vi "AlliGator Create Phasor Plot Additional Data String.vi"(6 "Average Plot Data (F)":bool, 7 "Include Header String (F)":bool, 8 "error in (no error)":errorcluster, 9 "Calibrated Phasor Plot":T2, 10 "Raw Phasor Plot":T4={"Phasor Plot Name"="", "Raw Phasor Plot"=[], "Phasor Frequency"=0.0, "[Decay Metadata]"=[], "Raw Phasor Plot SDV"=[], "Phasor SDV Options"={"Compute Estimated SDV"=FALSE, "# Replicas"=100, "Use Estimated Average Phasor"=FALSE}, "[Calibration Phasor]"=[]} {"[Decay Metadata]"."# Folds" min=1; "[Decay Metadata]"."ROI Descriptor"."Contours"."Type" items=["No Selection", "Point", "Line", "Rectangle", "Oval", "Polygon", "Freehand Region", "Annulus", "Unused2", "Unused3", "Broken Line", "Freehand Line", "Rotated Rectangle"]}, 11 "Phasor Plot Exported Data":T1) -> (0 "error out":errorcluster, 3 "Phasor Plot Additional Data String":string)   [LabVIEW 2021, in "AlliGator Phasor Graph.lvlib"]
doc: "Creates a string with all the user-requested phasor plot additional data."
uses:
  AlliGator Phasor Graph.lvlib
  AlliGator Raw Phasor Plot Data v4.ctl
  Phasor/Phasor (g, s).ctl
  AlliGator Decay Metadata v3.ctl
  AlliGator Decay Background Subtraction Info.ctl
  AlliGator Baseline Subtraction Method.ctl
  Graphs/XY Graph/XY Graph Plot Shift Parameters.ctl
  Graphs/XY Graph/XY Graph Plot Shift Method.ctl
  AlliGator Decay Extrapolation Parameters.ctl
  Phasor/Phasor Standard Deviation Options.ctl
  Phasor/Calibration Phasor (m, phi).ctl
  AlliGator Phasor Plot Additional Data List.ctl
  Graphs/XY Graph/XY Plot Data.ctl
  AlliGator Phasor Plot Exported Data Selection.ctl
  d5eb63e0-648c-47d6-be91-64ae69301d4e.vi
  28782bb2-77f9-4fec-b09f-3ba0b8238253.vi
  <userlib>/_OpenG.lib/array/array.llb/Filter 1D Array (DBL)__ogtk.vi
  Strings/Strings.lvlib
  Phasor/Phasor.lvlib
  AlliGator Phasor Ratio.lvlib
  Time/Time.lvlib
  <vilib>/Analysis/NI_AALBase.lvlib
  Utilities/Utilities.lvlib
  <userlib>/_OpenG.lib/array/array.llb/openg_array.lvlib
  AlliGator Decay Preprocessing.lvlib
  Graphs/XY Graph/XY Graph Add-Ons.lvlib
panel:
  out "CPU (s)":dbl
  in  "Phasor Plot Exported Data List":T3
  # "see the AlliGator License on the block diagram (Ctrl+E or Window:Show Block Diagram)"
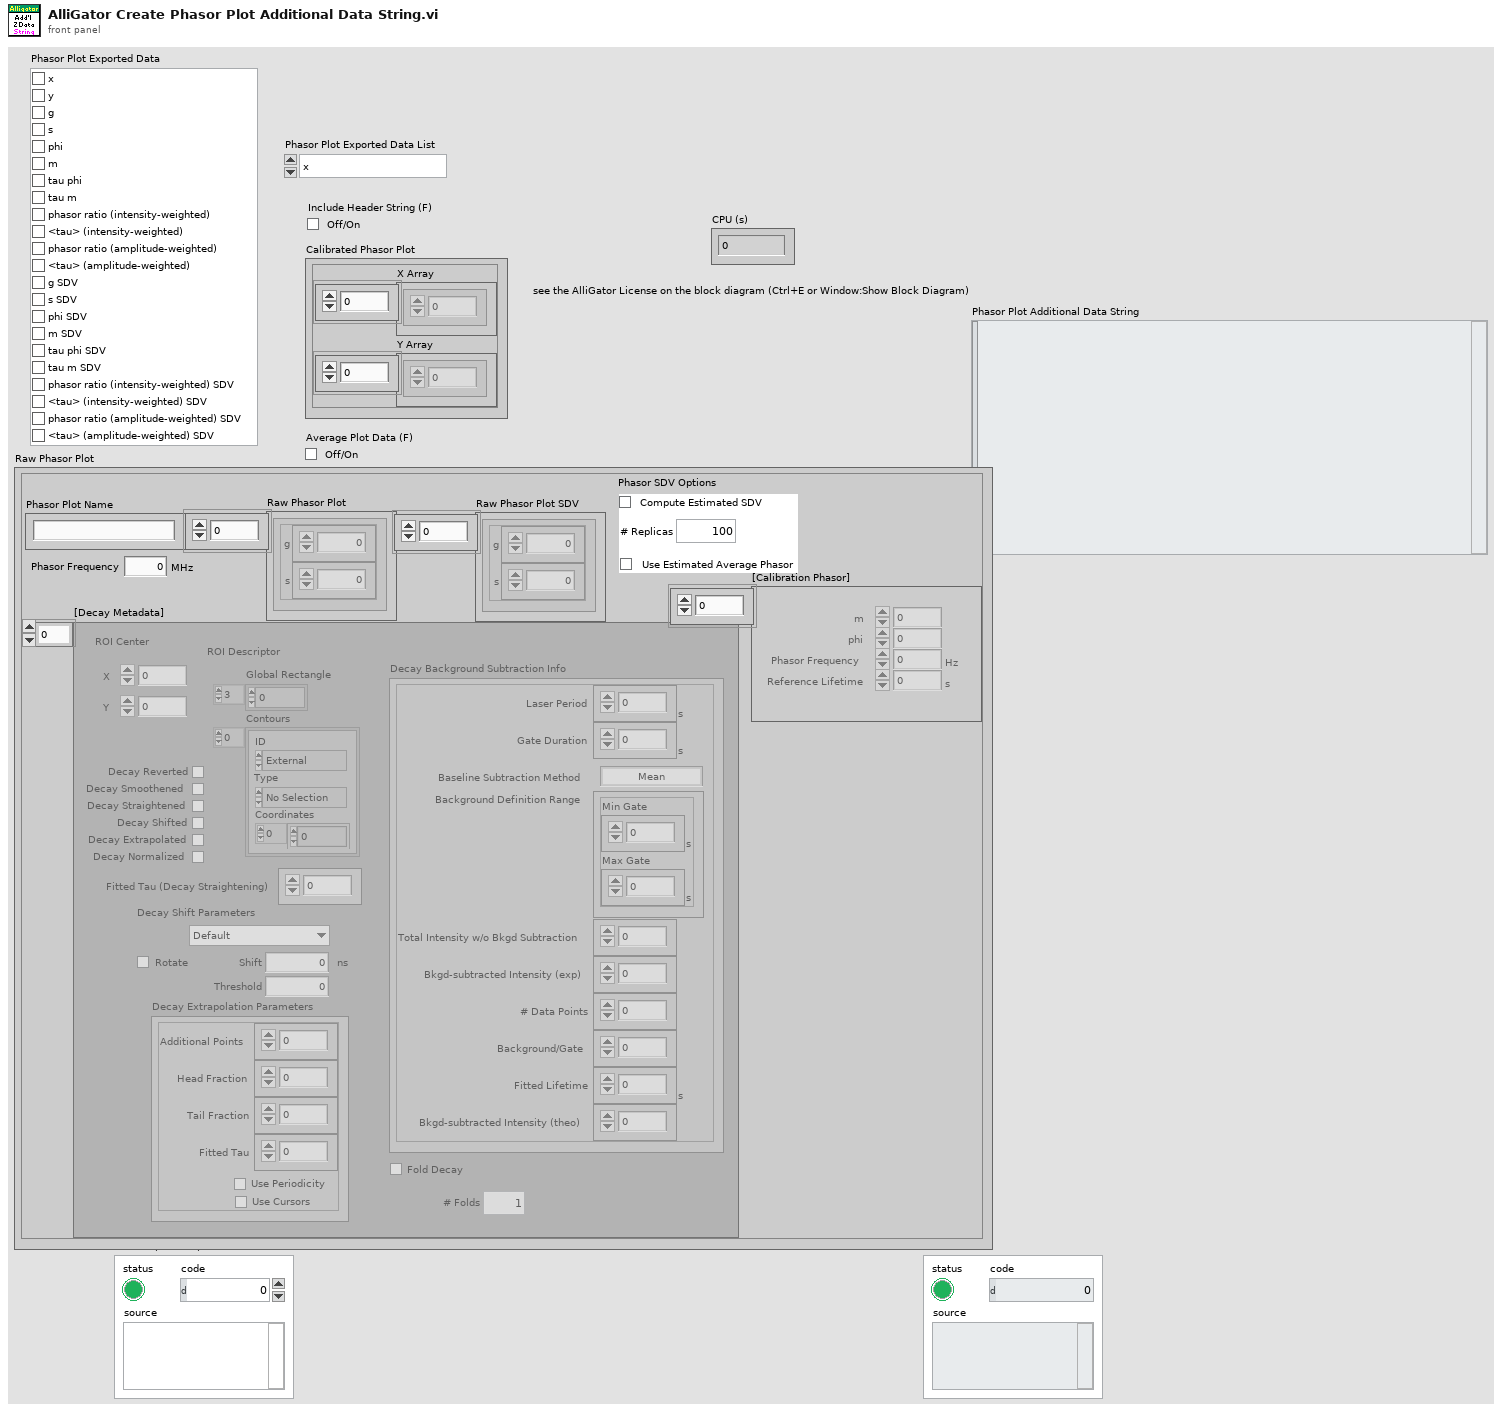
[diagram p1: front panel]
types:
  T1 = typedef "AlliGator Phasor Graph.lvlib/AlliGator Phasor Plot Exported Data Selection.ctl" = cluster{"x":bool, "y":bool, "g":bool, "s":bool, "phi":bool, "m":bool, "tau phi":bool, "tau m":bool, "phasor ratio (intensity-weighted)":bool, "<tau> (intensity-weighted)":bool, "phasor ratio (amplitude-weighted)":bool, "<tau> (amplitude-weighted)":bool, "g SDV":bool, "s SDV":bool, "phi SDV":bool, "m SDV":bool, "tau phi SDV":bool, "tau m SDV":bool, "phasor ratio (intensity-weighted) SDV":bool, "<tau> (intensity-weighted) SDV":bool, "phasor ratio (amplitude-weighted) SDV":bool, "<tau> (amplitude-weighted) SDV":bool}
  T2 = typedef "XY Graph Add-Ons.lvlib/XY Plot Data.ctl" = cluster{"X Array":dbl[], "Y Array":dbl[]}
  T3 = typedef "AlliGator Phasor Graph.lvlib/AlliGator Phasor Plot Additional Data List.ctl" = enum16{"x", "y", "g", "s", "phi", "m", "tau phi", "tau m", "phasor ratio (intensity-weighted)", "<tau> (intensity-weighted)", "phasor ratio (amplitude-weighted)", "<tau> (amplitude-weighted)", "g SDV", "s SDV", "phi SDV", "m SDV", "tau phi SDV", "tau m SDV", "phasor ratio (intensity-weighted) SDV", "<tau> (intensity-weighted) SDV", "phasor ratio (amplitude-weighted) SDV", "<tau> (amplitude-weighted) SDV"}
  T4 = typedef "AlliGator Phasor Graph.lvlib/AlliGator Raw Phasor Plot Data v4.ctl" = cluster{"Phasor Plot Name":string, "Raw Phasor Plot":T5[], "Phasor Frequency":dbl[unit], "[Decay Metadata]":T6[], "Raw Phasor Plot SDV":T5[], "Phasor SDV Options":T13, "[Calibration Phasor]":T14[]}
  T5 = typedef "Phasor.lvlib/Phasor (g, s).ctl" = cluster{"g":dbl, "s":dbl}
  T6 = typedef "AlliGator Phasor Graph.lvlib/AlliGator Decay Metadata v3.ctl" = cluster{"ROI Descriptor":T7, "ROI Center":cluster{"X":i32, "Y":i32}, "Decay Background Subtraction Info":T8, "Decay Reverted":bool, "Decay Smoothened":bool, "Decay Straightened":bool, "Fitted Tau (Decay Straightening)":dbl, "Decay Shift Parameters":T10, "Decay Shifted":bool, "Decay Extrapolated":bool, "Decay Extrapolation Parameters":T12, "Decay Normalized":bool, "Fold Decay":bool, "# Folds":u32}
  T7 = typedef "ROI Descriptor" = cluster{"Global Rectangle":i32[], "Contours":cluster{"ID":enum32{"External", "Internal"}, "Type":u32, "Coordinates":i32[]}[]}
  T8 = typedef "AlliGator Decay Analysis.lvlib/AlliGator Decay Preprocessing.lvlib/AlliGator Decay Background Subtraction Info.ctl" = cluster{"Laser Period":dbl[unit], "Gate Duration":dbl[unit], "Baseline Subtraction Method":T9, "Background Definition Range":cluster{"Min Gate":dbl[unit], "Max Gate":dbl[unit]}, "Total Intensity w/o Bkgd Subtraction":dbl, "Bkgd-subtracted Intensity (exp)":dbl, "# Data Points":i32, "Background/Gate":dbl, "Fitted Lifetime":dbl[unit], "Bkgd-subtracted Intensity (theo)":dbl}
  T9 = typedef "AlliGator Decay Analysis.lvlib/AlliGator Decay Preprocessing.lvlib/AlliGator Baseline Subtraction Method.ctl" = enum16{"Mean", "Min", "Square Gated Single-Exponential", "File", "Constant"}
  T10 = typedef "XY Graph Add-Ons.lvlib/XY Graph Plot Shift Parameters.ctl" = cluster{"Type":T11, "Shift":dbl[unit], "Threshold":dbl, "Rotate":bool}
  T11 = typedef "XY Graph Add-Ons.lvlib/XY Graph Plot Shift Method.ctl" = enum16{"Default", "CFD", "Threshold", "Cross-Correlation"}
  T12 = typedef "AlliGator Decay Analysis.lvlib/AlliGator Decay Preprocessing.lvlib/AlliGator Decay Extrapolation Parameters.ctl" = cluster{"Additional Points":u32, "Head Fraction":dbl, "Fitted Tau":dbl, "Use Periodicity":bool, "Use Cursors":bool, "Tail Fraction":dbl}
  T13 = typedef "Phasor.lvlib/Phasor Standard Deviation Options.ctl" = cluster{"Compute Estimated SDV":bool, "# Replicas":u32, "Use Estimated Average Phasor":bool}
  T14 = typedef "Phasor.lvlib/Calibration Phasor (m, phi).ctl" = cluster{"m":dbl, "phi":dbl, "Phasor Frequency":dbl[unit], "Reference Lifetime":dbl[unit]}
  T15 = cluster{"Numeric Control":dbl, "Numeric Control":dbl}[]
  T16 = typedef "Phasor.lvlib/Phasor (m, phi).ctl" = cluster{"m":dbl, "phi":dbl}
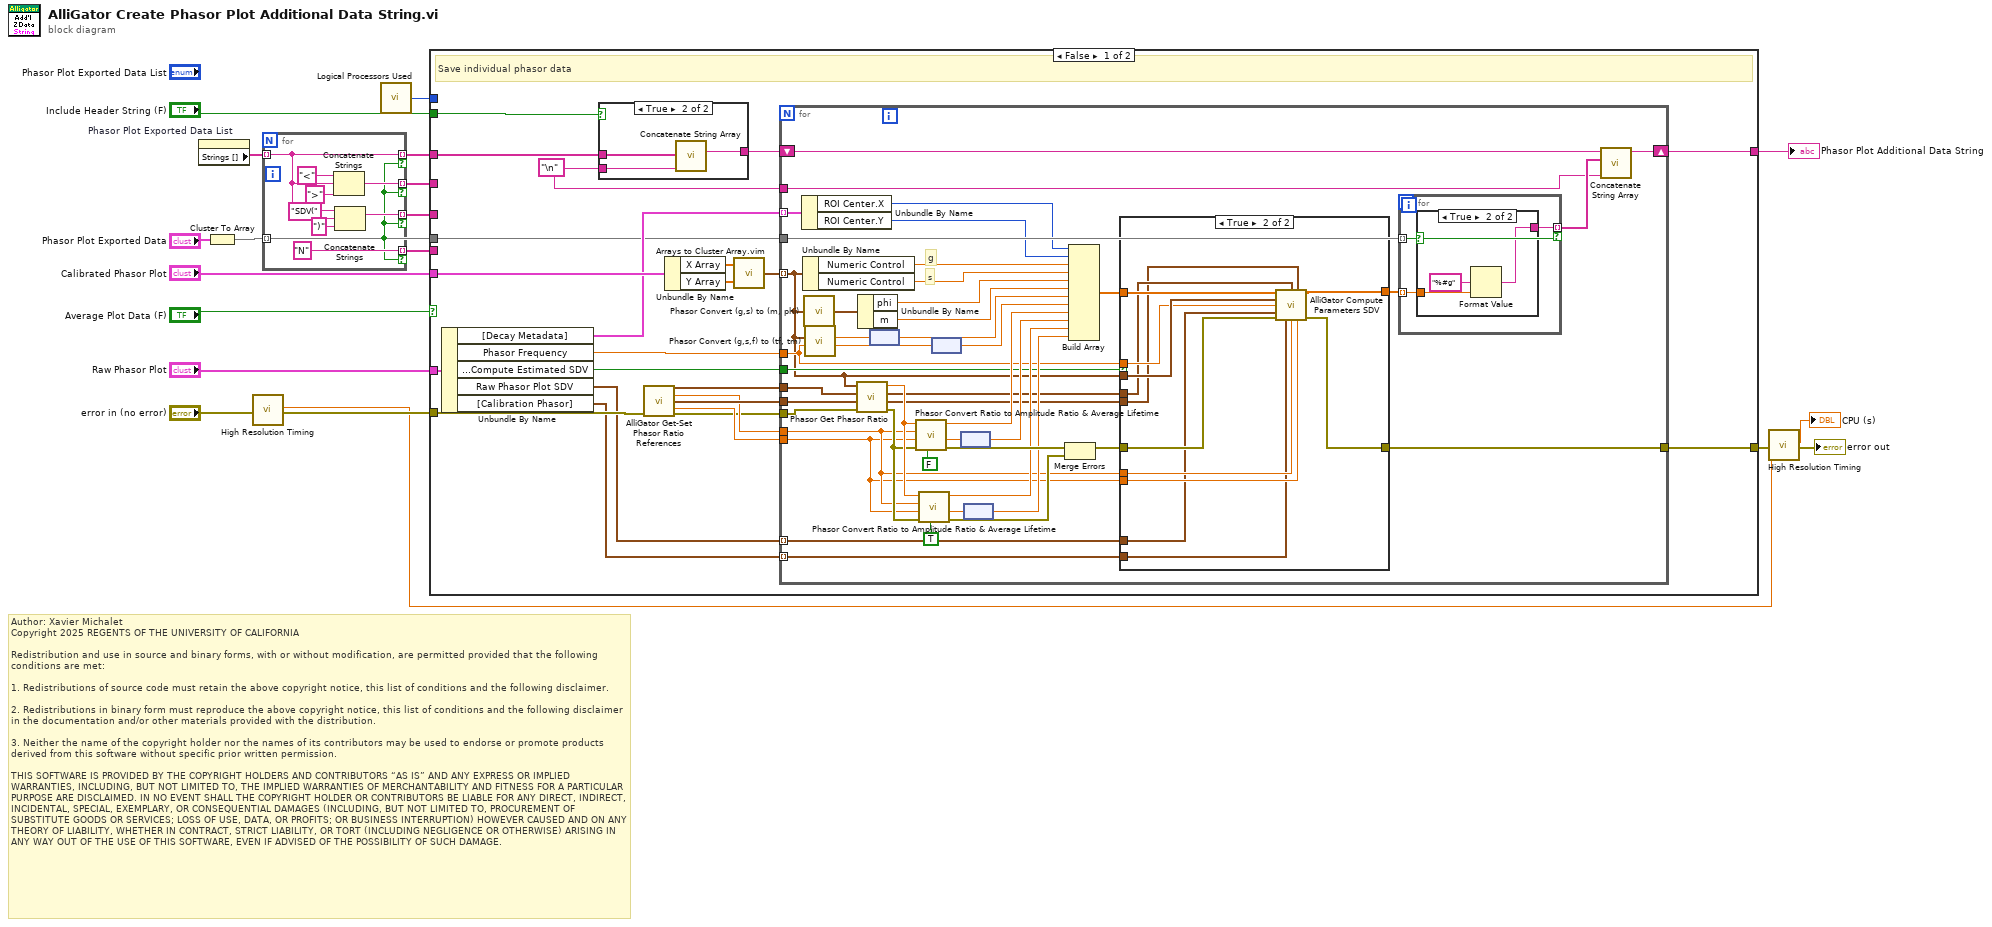
[diagram p0: block diagram]
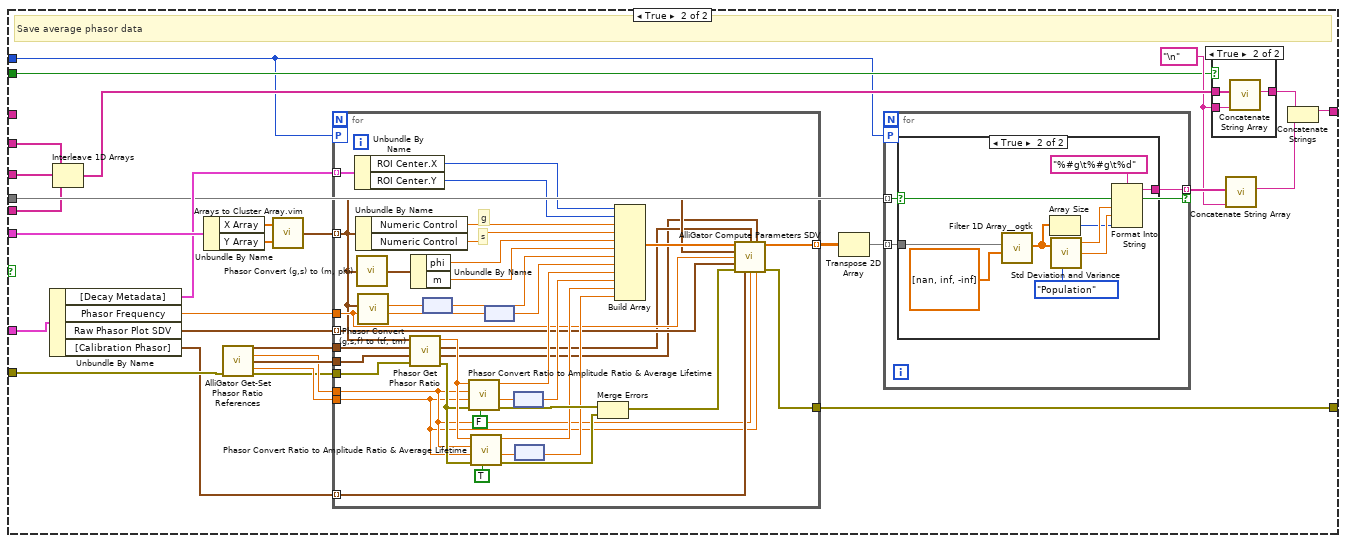
[diagram p5: hidden frame]
diagram:
  # "Author: Xavier Michalet\nCopyright 2025 REGENTS OF THE UNIVERSITY OF CALIFORNIA\n\nRedistribution and use in source and binary forms, with or without modification, are permitted provided that the following conditions are met:\n\n1. Redistributions of source code must retain the above copyright notice, this list of conditions and the following disclaimer.\n\n2. Redistributions in binary form must reproduce the above copyright notice, this list of conditions and the following disclaimer in the documentation and/or other materials provided with the distribution.\n\n3. Neither the name of the copyright holder nor the names of its contributors may be used to endorse or promote products derived from this software without specific prior written permission.\n\nTHIS SOFTWARE IS PROVIDED BY THE COPYRIGHT HOLDERS AND CONTRIBUTORS “AS IS” AND ANY EXPRESS OR IMPLIED WARRANTIES, INCLUDING, BUT NOT LIMITED TO, THE IMPLIED WARRANTIES OF MERCHANTABILITY AND FITNESS FOR A PARTICULAR PURPOSE ARE DISCLAIMED. IN NO EVENT SHALL THE COPYRIGHT HOLDER OR CONTRIBUTORS BE LIABLE FOR ANY DIRECT, INDIRECT, INCIDENTAL, SPECIAL, EXEMPLARY, OR CONSEQUENTIAL DAMAGES (INCLUDING, BUT NOT LIMITED TO, PROCUREMENT OF SUBSTITUTE GOODS OR SERVICES; LOSS OF USE, DATA, OR PROFITS; OR BUSINESS INTERRUPTION) HOWEVER CAUSED AND ON ANY THEORY OF LIABILITY, WHETHER IN CONTRACT, STRICT LIABILITY, OR TORT (INCLUDING NEGLIGENCE OR OTHERWISE) ARISING IN ANY WAY OUT OF THE USE OF THIS SOFTWARE, EVEN IF ADVISED OF THE POSSIBILITY OF SUCH DAMAGE."
  n1 = property on="Phasor Plot Exported Data List" class="Enum (strict)"() -> ("Strings []"=w19:string[])  [unwired: 2 in, 2 out]
  n2 = Cluster To Array(cluster="Phasor Plot Exported Data") -> (array=w13:bool[])
  n3 = call "High Resolution Timing.vi"("Error In"="error in (no error)") -> ("elapsed (relative) seconds"=w8:dbl, "Error Out"=w10:errorcluster)  [unwired: 16 in, 1 out]
  n4 = for {
    tunnel: w13 -> [w20] mode=indexing
    tunnel: w19 -> [w23] mode=indexing
    tunnel: [w23] -> w16 mode=indexing if=w20
    tunnel: [w26] -> w5 mode=indexing if=w20
    tunnel: [w25] -> w4 mode=indexing if=w20
    tunnel: ["N" ("string")] -> w2 mode=indexing if=w20
    n5 = Concatenate Strings("<" ("string"), w23, ">" ("string")) -> (w26:string)
    n6 = Concatenate Strings("SDV(" ("string"), w23, ")" ("string")) -> (w25:string)
  }
  n7 = call "Logical Processors Used.vi"() -> ("# Logical Processor Used"=w1:i32)  [unwired: 6 in]
  n8 = case shown="False" "Average Plot Data (F)" {
    tunnel: "Raw Phasor Plot" -> [w46 w147]
    tunnel: "Calibrated Phasor Plot" -> [w51 w151]
    tunnel: w16 -> [w47 _]
    tunnel: w10 -> [w39 w140]
    tunnel: w13 -> [w34 w132]
    tunnel: [w37 w127] -> w12
    tunnel: [w36 w139] -> w11
    tunnel: w5 -> [_ w137]
    tunnel: w4 -> [_ w136]
    tunnel: "Include Header String (F)" -> [w33 w126]
    tunnel: w2 -> [_ w125]
    tunnel: w1 -> [_ w124]
    frame False {
      w32 = "\n"
      # "Save individual phasor data"
      n9 = Unbundle By Name(w46) -> ("[Decay Metadata]"=w35:T6[], "Phasor Frequency"=w45:dbl[unit], "Phasor SDV Options.Compute Estimated SDV"=w29:bool, "Raw Phasor Plot SDV"=w31:T5[], "[Calibration Phasor]"=w30:T14[])
      n10 = case shown="True" w33 {
        tunnel: w47 -> [_ w54]
        tunnel: [_ w53] -> w38
        tunnel: w32 -> [_ w52]
        frame False {
        }
        frame True {
          n11 = call "Concatenate String Array.vi"("Suffix (\"\")"=w52, "String Array"=w54) -> ("Formatted String"=w53:string)  [unwired: 9 in]
        }
      }
      n12 = call "AlliGator Get-Set Phasor Ratio References.vi"("error in (no error)"=w39) -> ("Reference Phasor 1"=w44:T5, "Reference Lifetime 1"=w42:dbl[unit], "Reference Phasor 2"=w43:T5, "Reference Lifetime 2"=w41:dbl[unit], "error out"=w40:errorcluster)  [unwired: 7 in, 3 out]
      n13 = Unbundle By Name(w51) -> ("X Array"=w50:dbl[], "Y Array"=w49:dbl[])
      n14 = call "Arrays to Cluster Array.vim"("Array 1"=w50, "Array 2"=w49) -> ("Cluster Array"=w48:T15)  [unwired: 6 in]
      n15 = for {
        tunnel: w48 -> [w59] mode=indexing
        tunnel: w45 -> [w60]
        tunnel: w44 -> [w58]
        tunnel: w43 -> [w57]
        tunnel: w42 -> [w56]
        tunnel: w41 -> [w55]
        tunnel: w40 -> [w94]
        shift-right: [w81] -> w37
        shift-left: w38 -> [w82]
        tunnel: w34 -> [w84]
        tunnel: w32 -> [w80]
        tunnel: [w62] -> w36
        tunnel: w35 -> [w78] mode=indexing
        tunnel: w31 -> [w64] mode=indexing
        tunnel: w30 -> [w61] mode=indexing
        tunnel: w29 -> [w67]
        # "s"
        # "g"
        n16 = Unbundle By Name(w78) -> ("ROI Center.X"=w77:i32, "ROI Center.Y"=w76:i32)
        n17 = Unbundle By Name(w59) -> ("Numeric Control"=w92:dbl, "Numeric Control"=w91:dbl)
        n18 = call "Phasor Convert (g,s) to (m, phi).vi"("Phasor (g, s)"=w59) -> ("Phasor (m, phi)"=w97:T16)  [unwired: 8 in]
        n19 = call "Phasor Convert (g,s,f) to (tf, tm).vi"("Phasor Harmonic Frequency"=w60, "Phasor (g, s)"=w59) -> ("Modulus Lifetime"=w95:dbl[unit], "Phase Lifetime"=w96:dbl[unit])  [unwired: 7 in, 1 out]
        n20 = call "Phasor Get Phasor Ratio.vi"("Error In"=w94, "Reference Phasor 2"=w57, "Reference Phasor 1"=w58, "Phasor"=w59) -> ("Error Out"=w71:errorcluster, "Phasor Ratio (f1)"=w72:dbl)  [unwired: 5 in, 1 out]
        n21 = Unbundle By Name(w97) -> ("phi"=w90:dbl, "m"=w89:dbl)
        n22 = node(w96) -> (w88:dbl)
        n23 = call "Phasor Convert Ratio to Amplitude Ratio & Average Lifetime.vi"("Compute Amplitude Ratio"=FALSE, "error in (no error)"=w71, "Reference Lifetime 2"=w55, "Reference Lifetime 1"=w56, "Phasor Ratio (f1)"=w72) -> ("error out"=w79:errorcluster, "Average Lifetime"=w93:dbl[unit], "Phasor/Amplitude Ratio"=w86:dbl)  [unwired: 2 in, 2 out]
        n24 = call "Phasor Convert Ratio to Amplitude Ratio & Average Lifetime.vi"("Compute Amplitude Ratio"=TRUE, "error in (no error)"=w71, "Reference Lifetime 2"=w55, "Reference Lifetime 1"=w56, "Phasor Ratio (f1)"=w72) -> ("error out"=w68:errorcluster, "Average Lifetime"=w74:dbl[unit], "Phasor/Amplitude Ratio"=w70:dbl)  [unwired: 2 in, 2 out]
        n25 = node(w95) -> (w87:dbl)
        n26 = node(w93) -> (w85:dbl)
        n27 = node(w74) -> (w69:dbl)
        n28 = Merge Errors(w79, w68) -> (w63:errorcluster)
        n29 = Build Array(w77, w76, w92, w91, w90, w89, w88, w87, w86, w85, w70, w69) -> (w66:dbl[])
        n30 = case shown="True" w67 {
          tunnel: w66 -> [w103 w115]
          tunnel: [w102 w114] -> w65
          tunnel: w64 -> [_ w109]
          tunnel: w63 -> [w98 w112]
          tunnel: [w98 w113] -> w62
          tunnel: w61 -> [_ w104]
          tunnel: w60 -> [_ w107]
          tunnel: w59 -> [_ w108]
          tunnel: w58 -> [_ w106]
          tunnel: w57 -> [_ w105]
          tunnel: w56 -> [_ w111]
          tunnel: w55 -> [_ w110]
          frame False {
            # "no SDV estimated"
            n31 = Initialize Array(0.0 ("Numeric Control"), 10 ("dimension size")) -> (w101:dbl[])
            n32 = Build Array (concatenate)(w103, w101) -> (w102:dbl[])
          }
          frame True {
            n33 = call "AlliGator Compute Parameters SDV.vi"("Parameters in"=w115, "Reference Phasor 1"=w106, "Reference Phasor 2"=w105, "Phasor"=w108, "Phasor Frequency"=w107, "Raw Phasor SDV"=w109, "error in (no error)"=w112, "Calibration Phasor"=w104, "Reference Lifetime 1"=w111, "Reference Lifetime 2"=w110) -> ("Parameters out"=w114:dbl[], "error out"=w113:errorcluster)  [unwired: 4 in]
          }
        }
        n34 = for {
          tunnel: w84 -> [w116] mode=indexing
          tunnel: w65 -> [w118] mode=indexing
          tunnel: [w117] -> w83 mode=indexing if=w116
          n35 = case shown="True" w116 {
            tunnel: w118 -> [_ w121]
            tunnel: [_ w119] -> w117
            frame False {
            }
            frame True {
              n36 = Format Value(format string="%#g", value (0)=w121) -> (output string=w119:string)  [unwired: 1 in]
            }
          }
        }
        n37 = call "Concatenate String Array.vi"("Suffix (\"\")"=w80, "String Array"=w83, "Prefix (\"\")"=w82) -> ("Formatted String"=w81:string)  [unwired: 8 in]
      }
    }
    frame True {
      w130 = "\n"
      # "Save average phasor data"
      n38 = Unbundle By Name(w147) -> ("[Decay Metadata]"=w138:T6[], "Phasor Frequency"=w146:dbl[unit], "Raw Phasor Plot SDV"=w123:T5[], "[Calibration Phasor]"=w122:T14[])
      n39 = Interleave 1D Arrays(w137, w136, w125) -> (w135:string[])
      n40 = Unbundle By Name(w151) -> ("X Array"=w150:dbl[], "Y Array"=w149:dbl[])
      n41 = call "AlliGator Get-Set Phasor Ratio References.vi"("error in (no error)"=w140) -> ("Reference Phasor 1"=w145:T5, "Reference Lifetime 1"=w143:dbl[unit], "Reference Phasor 2"=w144:T5, "Reference Lifetime 2"=w142:dbl[unit], "error out"=w141:errorcluster)  [unwired: 7 in, 3 out]
      n42 = call "Arrays to Cluster Array.vim"("Array 1"=w150, "Array 2"=w149) -> ("Cluster Array"=w148:T15)  [unwired: 6 in]
      n43 = for {
        tunnel: w148 -> [w173] mode=indexing
        tunnel: w146 -> [w174]
        tunnel: w145 -> [w171]
        tunnel: w144 -> [w170]
        tunnel: w143 -> [w168]
        tunnel: w142 -> [w167]
        tunnel: w141 -> [w200]
        tunnel: [w175] -> w139
        tunnel: w138 -> [w189] mode=indexing
        tunnel: [w177] -> w134 mode=indexing
        workers-P: w124 -> [_]
        tunnel: w123 -> [w172] mode=indexing
        tunnel: w122 -> [w169] mode=indexing
        # "s"
        # "g"
        n44 = Unbundle By Name(w189) -> ("ROI Center.X"=w188:i32, "ROI Center.Y"=w187:i32)
        n45 = Unbundle By Name(w173) -> ("Numeric Control"=w198:dbl, "Numeric Control"=w197:dbl)
        n46 = call "Phasor Convert (g,s) to (m, phi).vi"("Phasor (g, s)"=w173) -> ("Phasor (m, phi)"=w203:T16)  [unwired: 8 in]
        n47 = call "Phasor Convert (g,s,f) to (tf, tm).vi"("Phasor Harmonic Frequency"=w174, "Phasor (g, s)"=w173) -> ("Modulus Lifetime"=w201:dbl[unit], "Phase Lifetime"=w202:dbl[unit])  [unwired: 7 in, 1 out]
        n48 = call "Phasor Get Phasor Ratio.vi"("Error In"=w200, "Reference Phasor 2"=w170, "Reference Phasor 1"=w171, "Phasor"=w173) -> ("Error Out"=w180:errorcluster, "Phasor Ratio (f1)"=w185:dbl)  [unwired: 5 in, 1 out]
        n49 = Unbundle By Name(w203) -> ("phi"=w196:dbl, "m"=w195:dbl)
        n50 = node(w202) -> (w194:dbl)
        n51 = call "Phasor Convert Ratio to Amplitude Ratio & Average Lifetime.vi"("Compute Amplitude Ratio"=FALSE, "error in (no error)"=w180, "Reference Lifetime 2"=w167, "Reference Lifetime 1"=w168, "Phasor Ratio (f1)"=w185) -> ("error out"=w190:errorcluster, "Average Lifetime"=w199:dbl[unit], "Phasor/Amplitude Ratio"=w192:dbl)  [unwired: 2 in, 2 out]
        n52 = call "Phasor Convert Ratio to Amplitude Ratio & Average Lifetime.vi"("Compute Amplitude Ratio"=TRUE, "error in (no error)"=w180, "Reference Lifetime 2"=w167, "Reference Lifetime 1"=w168, "Phasor Ratio (f1)"=w185) -> ("error out"=w179:errorcluster, "Average Lifetime"=w183:dbl[unit], "Phasor/Amplitude Ratio"=w182:dbl)  [unwired: 2 in, 2 out]
        n53 = node(w201) -> (w193:dbl)
        n54 = node(w199) -> (w191:dbl)
        n55 = node(w183) -> (w181:dbl)
        n56 = Merge Errors(w190, w179) -> (w176:errorcluster)
        n57 = Build Array(w188, w187, w198, w197, w196, w195, w194, w193, w192, w191, w182, w181) -> (w178:dbl[])
        n58 = call "AlliGator Compute Parameters SDV.vi"("Parameters in"=w178, "Reference Phasor 1"=w171, "Reference Phasor 2"=w170, "Phasor"=w173, "Phasor Frequency"=w174, "Raw Phasor SDV"=w172, "error in (no error)"=w176, "Calibration Phasor"=w169, "Reference Lifetime 1"=w168, "Reference Lifetime 2"=w167) -> ("Parameters out"=w177:dbl[], "error out"=w175:errorcluster)  [unwired: 4 in]
      }
      n59 = Transpose 2D Array(2D array=w134) -> (transposed array=w133:dbl[][])
      n60 = for {
        tunnel: w133 -> [w157] mode=indexing
        tunnel: w132 -> [w155] mode=indexing
        tunnel: [w156] -> w131 mode=indexing if=w155
        workers-P: w124 -> [_]
        n61 = case shown="True" w155 {
          tunnel: w157 -> [_ w161]
          tunnel: [_ w162] -> w156
          frame False {
          }
          frame True {
            n62 = call-poly <userlib>:"Filter 1D Array__ogtk.vi"("items to filter"=dbl[] [nan, inf, -inf] ("Element(s) to Remove"), "array"=w161) -> ("filtered array"=w159:dbl[])  [unwired: 4 in, 1 out]
            n63 = Array Size(array=w159) -> (size(s)=w158:i32)
            n64 = call <vilib>:"Std Deviation and Variance.vi"("X"=w159, "Weighting (Sample)"=enum16{"Sample", "Population"}."Population") -> ("mean"=w165:dbl, "standard deviation"=w164:dbl)  [unwired: 1 out]
            n65 = Format Into String(format string="%#g\t%#g\t%d", w165, w164, w158) -> (resulting string=w162:string)  [unwired: 2 in, 1 out]
          }
        }
      }
      n66 = case shown="True" w126 {
        tunnel: w135 -> [_ w154]
        tunnel: w130 -> [_ w153]
        tunnel: [_ w152] -> w129
        frame False {
        }
        frame True {
          n67 = call "Concatenate String Array.vi"("Suffix (\"\")"=w153, "String Array"=w154) -> ("Formatted String"=w152:string)  [unwired: 9 in]
        }
      }
      n68 = call "Concatenate String Array.vi"("Suffix (\"\")"=w130, "String Array"=w131) -> ("Formatted String"=w128:string)  [unwired: 9 in]
      n69 = Concatenate Strings(w129, w128) -> (w127:string)
    }
  }
  "Phasor Plot Additional Data String" <- w12
  n70 = call "High Resolution Timing.vi"("relative seconds (NaN)"=w8, "Error In"=w11) -> ("elapsed (relative) seconds"=→"CPU (s)":dbl, "Error Out"=→"error out":errorcluster)  [unwired: 15 in, 1 out]
